vi "Set_para_port0.vi"(8 "error in (no error)":errorcluster caption="错误输入（无错误）", 10 "R or W":enum16{"read", "write"}(ring), 11 "address":i16=888 caption="地址" format="%.0x") -> (0 "error out":errorcluster caption="错误输出", 3 "address 2":i16=888 caption="地址" format="%.0x")   [LabVIEW 2011]
uses:
  <vilib>/Platform/portaccess.llb/In Port8.vi
  <vilib>/Platform/portaccess.llb/Out Port32.vi
panel:
  out "Control":i16=888 caption="控制" format="%.0x"
  out "Status":i16=888 caption="状态" format="%.0x"
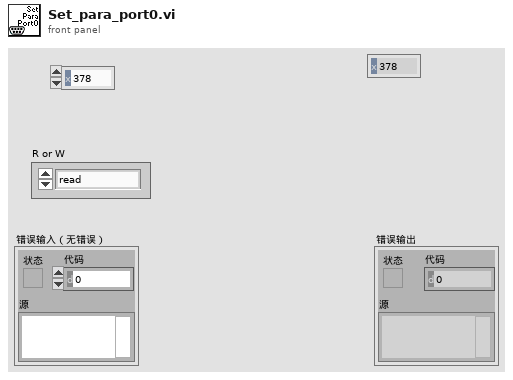
[diagram p1: front panel]
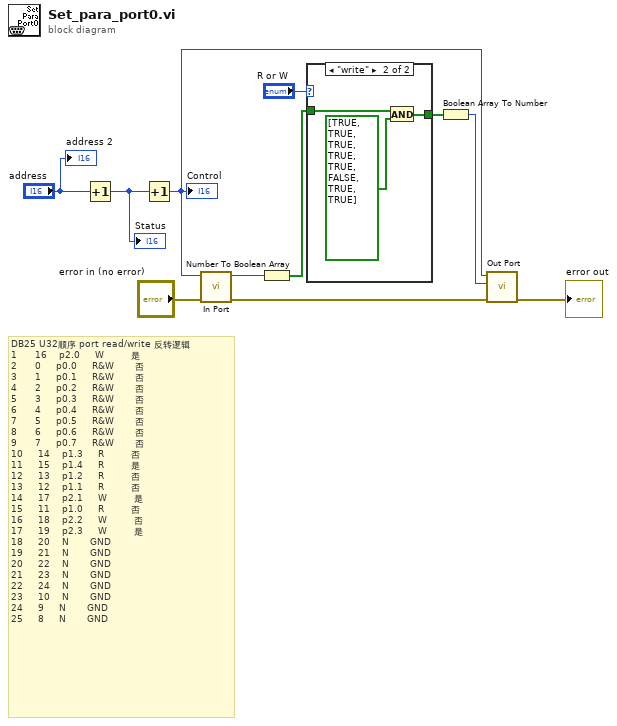
[diagram p0: block diagram]
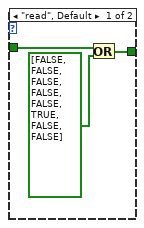
[diagram p2: hidden frame]
diagram:
  # "DB25\tU32顺序\tport\tread/write\t反转逻辑\n1\t     16\t   p2.0    \tW\t        是\n2\t     0    \tp0.0\t   \tR&W\t      否\n3\t     1\t\t   p0.1\t   \tR&W      \t否\n4\t\t    2\t   \tp0.2   \t\tR&W      \t否\n5\t\t    3\t\t   p0.3   \t\tR&W\t      否\n6\t\t    4\t   \tp0.4   \t\tR&W      \t否\n7\t\t    5\t   \tp0.5   \t\tR&W      \t否\n8\t\t    6\t   \tp0.6\t   \tR&W      \t否\n9\t    \t7\t   \tp0.7\t   \tR&W\t      否\n10\t    14   \tp1.3   \t\tR        \t否\n11\t   \t15   \tp1.4   \t\tR        \t是\n12\t   \t13   \tp1.2\t   \tR        \t否\n13    \t12   \tp1.1\t   \tR        \t否\n14     17   \tp2.1\t   \tW        \t是\n15    \t11   \tp1.0   \t\tR\t        否\n16    \t18   \tp2.2   \t\tW        \t否\n17    \t19\t   p2.3   \t\tW\t        是\n18    \t20   \tN   \t  \tGND\t\n19    \t21   \tN   \t  \tGND\t\n20\t    22\t   N\t  \t  \tGND\t\n21\t    23\t   N  \t  \t\tGND\t\n22\t    24\t   N  \t  \t\tGND\t\n23    \t10   \tN  \t  \t\tGND\t\n24    \t9\t    N  \t  \t\tGND\t\n25\t    8    \tN  \t  \t\tGND"
  n1 = Increment(x="address") -> (x+1=w11:i16)
  "Status" <- w11
  n2 = Increment(x=w11) -> (x+1=w10:i16)
  "Control" <- w10
  n3 = call-poly <vilib>:"In Port.vi"("error in (no error)"="error in (no error)", "address"=w10) -> ("error out"=w8:errorcluster, "data read"=w9:i8)  [unwired: 6 in]
  n4 = Number To Boolean Array(number=w9) -> (Boolean array=w7:bool[])
  n5 = case shown="\"write\"" "R or W" {
    tunnel: w7 -> [w14 w17]
    tunnel: [w12 w15] -> w6
    frame "read", Default {
      n6 = Or(x=w14, y=bool[] [FALSE, FALSE, FALSE, FALSE, FALSE, TRUE, FALSE, FALSE]) -> (x .or. y?=w12:bool[])
    }
    frame "write" {
      n7 = And(x=w17, y=bool[] [TRUE, TRUE, TRUE, TRUE, TRUE, FALSE, TRUE, TRUE]) -> (x .and. y?=w15:bool[])
    }
  }
  n8 = Boolean Array To Number(Boolean array=w6) -> (number=w5:u32)
  n9 = call-poly <vilib>:"Out Port.vi"("error in (no error)"=w8, "write value"=w5, "address"=w10) -> ("error out"=→"error out":errorcluster)  [unwired: 6 out]
  "address 2" <- "address"
